vi "Manipulator Move Rel Abs.vi"(8 "error in (no error)":errorcluster, 9 "ABS":bool, 10 "Deltas":cluster{"X":i32, "Y":i32, "Z":i32}, 11 "VISA resource in":refnum<visa-resource-name>="COM1") -> (0 "error out":errorcluster, 2 "Response":string, 3 "VISA resource out":refnum<visa-resource-name>)   [LabVIEW 2012, in "Scientifica Manipulator Daemon.lvlib"]
uses:
  Scientifica Manipulator Daemon.lvlib
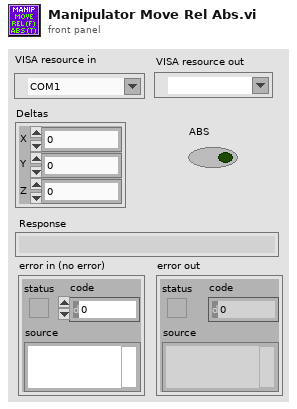
[diagram p1: front panel]
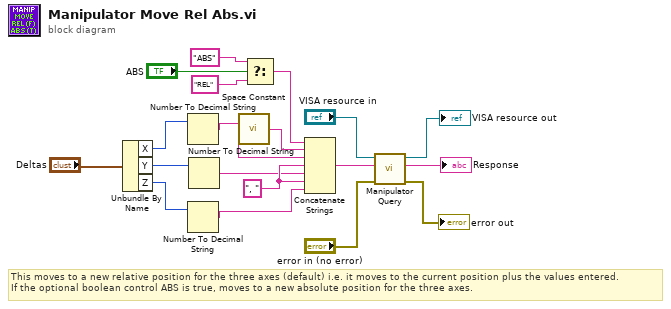
[diagram p0: block diagram]
diagram:
  w9 = ", " ("string")
  # "This moves to a new relative position for the three axes (default) i.e. it moves to the current position plus the values entered.\nIf the optional boolean control ABS is true, moves to a new absolute position for the three axes."
  n1 = Unbundle By Name("Deltas") -> ("X"=w7:i32, "Y"=w6:i32, "Z"=w5:i32)
  n2 = Number To Decimal String(number=w7) -> (decimal integer string=w4:string)  [unwired: 1 in]
  n3 = Number To Decimal String(number=w5) -> (decimal integer string=w2:string)  [unwired: 1 in]
  n4 = Number To Decimal String(number=w6) -> (decimal integer string=w3:string)  [unwired: 1 in]
  n5 = call <vilib>:"Space Constant.vi"() -> ("String"=w10:string)
  n6 = Select(t="ABS", s="ABS", f="REL") -> (s? t:f=w11:string)
  n7 = Concatenate Strings(w11, w10, w4, w9, w3, w9, w2) -> (w8:string)
  n8 = call "Manipulator Query.vi"("error in (no error)"="error in (no error)", "Command"=w8, "VISA resource in"="VISA resource in") -> ("error out"=→"error out":errorcluster, "Response"=→"Response":string, "VISA resource out"=→"VISA resource out":refnum<visa-resource-name>)  [unwired: 5 in, 1 out]
